vi "(SubVI) Three Axises Move to MiddlePI_YCC.vi"   [LabVIEW 2014]
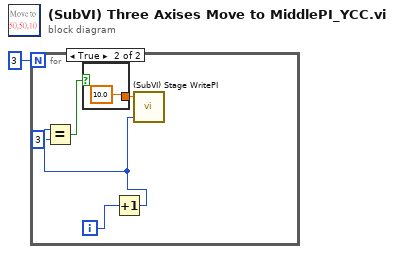
[diagram p0: block diagram]
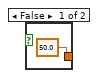
[diagram p2: hidden frame]
diagram:
  n1 = for {
    N: 3 -> [_]
    i -> [w6]
    n2 = Increment(x=w6) -> (x+1=w3:i32)
    n3 = Equal?(x=w3, y=3) -> (x = y?=w4:bool)
    n4 = case shown="True" w4 {
      tunnel: [50.0 ("position") 10.0 ("position")] -> w5
      frame False {
      }
      frame True {
      }
    }
    n5 = call "(SubVI) Stage WritePI.vi"("axis"=w3, "position"=w5) -> ()  [unwired: 4 in]
  }
